vi "GenerateTextFragments.vi"(8 "error in (no error)":errorcluster, 9 "textPosition in":u32, 10 "textFragment in":T1, 11 "xmlelement in":refnum<k20>) -> (0 "error out":errorcluster, 1 "textPosition out":u32, 2 "textFragments out":T1[](array[typedef]), 3 "xmlelement out":refnum<k20>)   [LabVIEW 2010, in "StyledText.lvlib"]
doc: "Generates text fragments from the given XML node. Uses recursion to read child nodes.\n\nCopyright (c) 2018, Martin Weiss\nAll rights reserved.\n\nRedistribution and use in source and binary forms, with or without modification, are permitted provided that the following conditions are met:\n\n1. Redistributions of source code must retain the above copyright notice, this list of conditions and the following disclaimer.\n\n2. Redistributions in binary form must reproduce the above copyright notice, this list of conditions and the following disclaimer in the documentation and/or other materials provided with the distribution.\n\nTHIS SOFTWARE IS PROVIDED BY THE COPYRIGHT HOLDERS AND CONTRIBUTORS \"AS IS\" AND ANY EXPRESS OR IMPLIED WARRANTIES, INCLUDING, BUT NOT LIMITED TO, THE IMPLIED WARRANTIES OF MERCHANTABILITY AND FITNESS FOR A PARTICULAR PURPOSE ARE DISCLAIMED. IN NO EVENT SHALL THE COPYRIGHT HOLDER OR CONTRIBUTORS BE LIABLE FOR ANY DIRECT, INDIRECT, INCIDENTAL, SPECIAL, EXEMPLARY, OR CONSEQUENTIAL DAMAGES (INCLUDING, BUT NOT LIMITED TO, PROCUREMENT OF SUBSTITUTE GOODS OR SERVICES; LOSS OF USE, DATA, OR PROFITS; OR BUSINESS INTERRUPTION) HOWEVER CAUSED AND ON ANY THEORY OF LIABILITY, WHETHER IN CONTRACT, STRICT LIABILITY, OR TORT (INCLUDING NEGLIGENCE OR OTHERWISE) ARISING IN ANY WAY OUT OF THE USE OF THIS SOFTWARE, EVEN IF ADVISED OF THE POSSIBILITY OF SUCH DAMAGE."
uses:
  StyledText.lvlib
  TextFragment.ctl
  <vilib>/Utility/miscctls.llb/LVSelectionTypeDef.ctl
  <vilib>/Utility/miscctls.llb/LVFontTypeDef.ctl
  <vilib>/xml/Close Reference(Node).vi
  Program Files (x86)/National Instruments/LabVIEW 2010/resource/objmgr/DOMUserDefRef.rc
  <vilib>/xml/NI_XML.lvlib
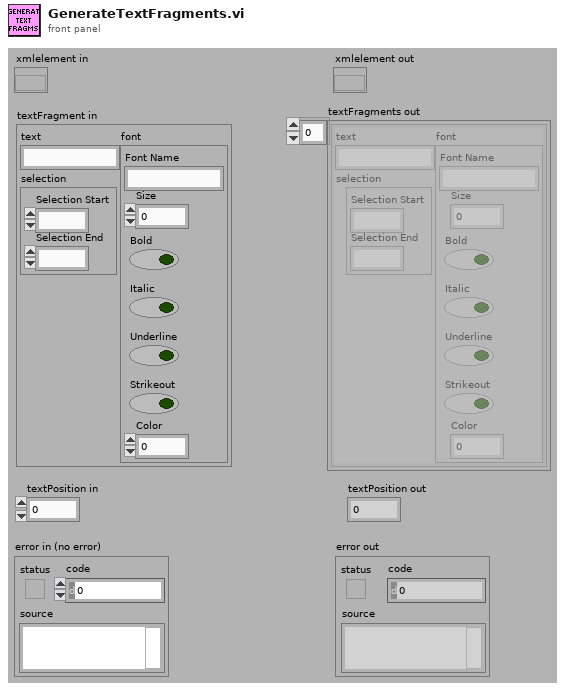
[diagram p1: front panel]
types:
  T1 = typedef "StyledText.lvlib/TextFragment.ctl" = cluster{"text":string, "selection":T2, "font":T3}
  T2 = typedef "LVSelectionTypeDef.ctl" = cluster{"Selection Start":u32, "Selection End":u32}
  T3 = typedef "LVFontTypeDef.ctl" = cluster{"Font Name":string, "Size":u16, "Bold":bool, "Italic":bool, "Underline":bool, "Strikeout":bool, "Color":u32}
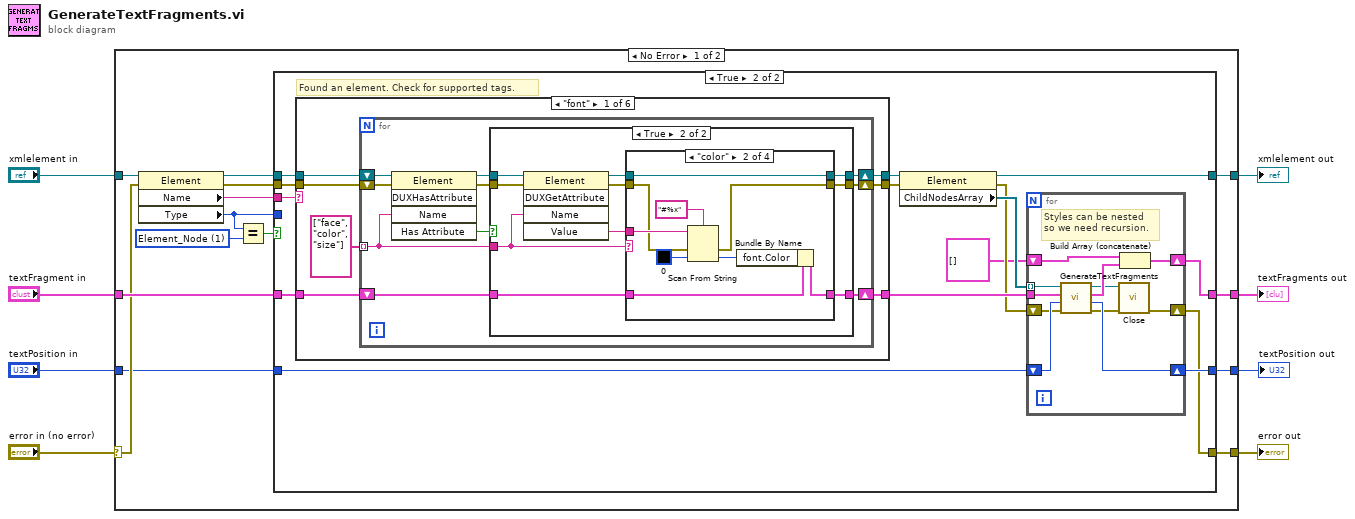
[diagram p0: block diagram]
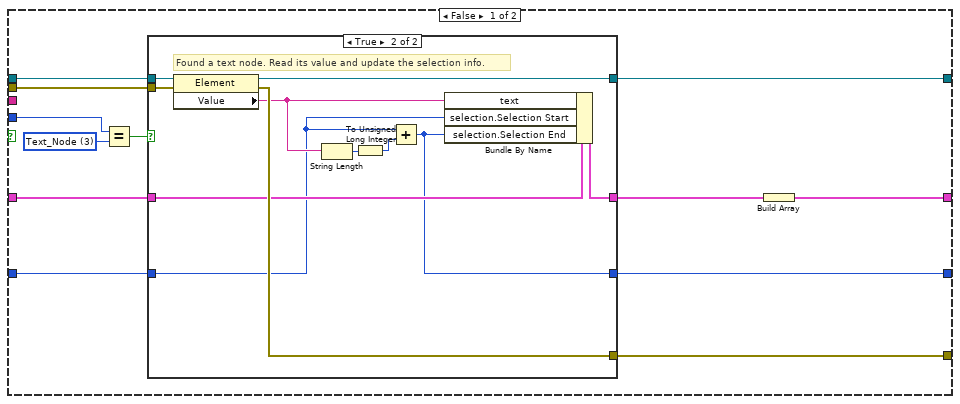
[diagram p2: hidden frame]
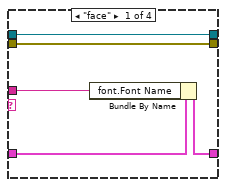
[diagram p5: hidden frame]
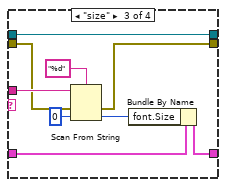
[diagram p6: hidden frame]
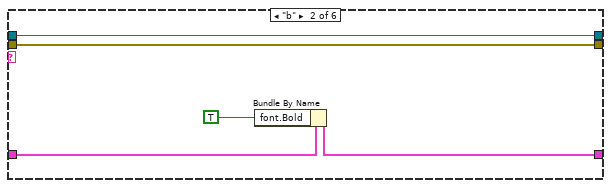
[diagram p8: hidden frame]
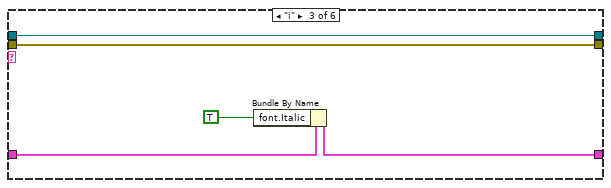
[diagram p9: hidden frame]
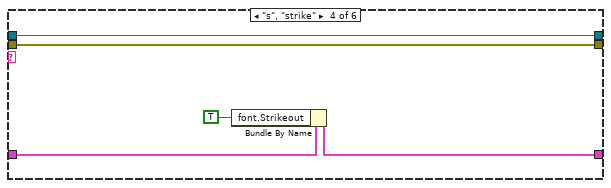
[diagram p10: hidden frame]
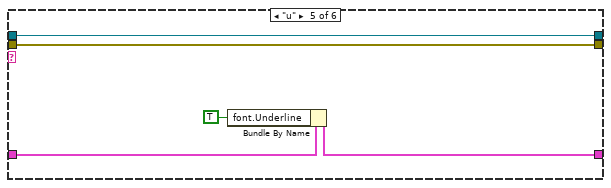
[diagram p11: hidden frame]
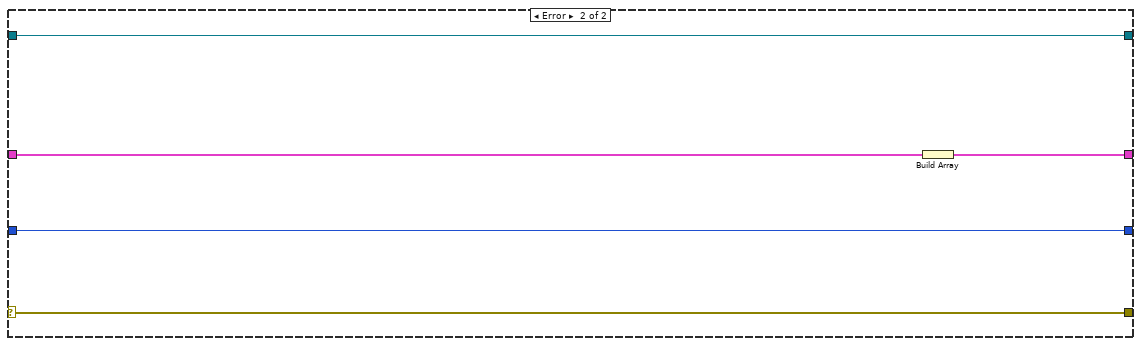
[diagram p13: hidden frame]
diagram:
  n1 = case shown="No Error" "error in (no error)" {
    selector: "error in (no error)" -> [w18 w158]
    tunnel: "textFragment in" -> [w22 w159]
    tunnel: [w21 w155] -> w7
    tunnel: "xmlelement in" -> [w20 w157]
    tunnel: [w15 w158] -> w4
    tunnel: [w11 w157] -> w3
    tunnel: "textPosition in" -> [w10 w156]
    tunnel: [w9 w156] -> w1
    frame No Error {
      w14 = 1 items=["Element_Node"=1, "Attribute_Node"=2, "Text_Node"=3, "CDATASection_Node"=4, "EntityReference_Node"=5, "Entity_Node"=6, "ProcessingInstruction_Node"=7, "Comment_Node"=8, "Document_Node"=9, "DocumentType_Node"=10, "DocumentFragment_Node"=11, "Notation_Node"=12] ("Node Type")
      n2 = property class="Element"(reference=w20, error in=w18) -> (reference out=w19:refnum<k20>, error out=w16:errorcluster, "Name"=w17:string, "Type"=w12:i32)
      n3 = Equal?(x=w12, y=w14) -> (x = y?=w13:bool)
      n4 = case shown="True" w13 {
        tunnel: w22 -> [w30 w64]
        tunnel: [w23 w52] -> w21
        tunnel: w19 -> [w31 w63]
        tunnel: w17 -> [_ w62]
        tunnel: w16 -> [w28 w61]
        tunnel: [w27 w50] -> w15
        tunnel: w12 -> [w33 _]
        tunnel: [w26 w59] -> w11
        tunnel: w10 -> [w25 w58]
        tunnel: [w24 w57] -> w9
        frame False {
          w34 = 3 items=["Element_Node"=1, "Attribute_Node"=2, "Text_Node"=3, "CDATASection_Node"=4, "EntityReference_Node"=5, "Entity_Node"=6, "ProcessingInstruction_Node"=7, "Comment_Node"=8, "Document_Node"=9, "DocumentType_Node"=10, "DocumentFragment_Node"=11, "Notation_Node"=12] ("Node Type")
          n5 = Equal?(x=w33, y=w34) -> (x = y?=w32:bool)
          n6 = case shown="True" w32 {
            tunnel: w31 -> [w36 w49]
            tunnel: w30 -> [w38 w44]
            tunnel: [w38 w43] -> w29
            tunnel: w28 -> [w37 w48]
            tunnel: [w37 w47] -> w27
            tunnel: [w36 w46] -> w26
            tunnel: w25 -> [w35 w42]
            tunnel: [w35 w41] -> w24
            frame False {
            }
            frame True {
              # "Found a text node. Read its value and update the selection info."
              n7 = property class="Element"(reference=w49, error in=w48) -> (reference out=w46:refnum<k20>, error out=w47:errorcluster, "Value"=w45:string)
              n8 = String Length(string=w45) -> (length=w40:i32)
              n9 = To Unsigned Long Integer(number=w40) -> (unsigned 32bit integer=w39:u32)
              n10 = Add(x=w42, y=w39) -> (x+y=w41:u32)
              n11 = Bundle By Name(cluster=w44, "text"=w45, "selection.Selection Start"=w42, "selection.Selection End"=w41) -> (w43:T1)
            }
          }
          n12 = Build Array(w29) -> (w23:T1[])
        }
        frame True {
          # "Found an element. Check for supported tags."
          n13 = case shown="\"font\"" w62 {
            tunnel: w63 -> [w78 w133 w138 w143 w148 w152]
            tunnel: [w82 w136 w141 w146 w151 w154] -> w60
            tunnel: w64 -> [w81 w134 w139 w144 w149 w154]
            tunnel: w61 -> [w80 w135 w140 w145 w150 w153]
            tunnel: [w79 w135 w140 w145 w150 w153] -> w55
            tunnel: [w77 w133 w138 w143 w148 w152] -> w56
            frame "font" {
              n14 = for {
                shift-right: [w87] -> w82
                shift-left: w81 -> [w86]
                shift-right: [w84] -> w79
                shift-left: w80 -> [w92]
                shift-right: [w85] -> w77
                shift-left: w78 -> [w90]
                tunnel: string[] ["face", "color", "size"] -> [w83] mode=indexing
                n15 = invoke class="Element" method="DUXHasAttribute"(reference=w90, error in=w92, "Name"=w83) -> (reference out=w89:refnum<k20>, error out=w91:errorcluster, "Has Attribute"=w88:bool)  [unwired: 2 in, 2 out]
                n16 = case shown="True" w88 {
                  tunnel: w91 -> [w94 w105]
                  tunnel: w89 -> [w95 w104]
                  tunnel: [w93 w102] -> w87
                  tunnel: w86 -> [w93 w101]
                  tunnel: [w95 w99] -> w85
                  tunnel: [w94 w97] -> w84
                  tunnel: w83 -> [_ w96]
                  frame False {
                  }
                  frame True {
                    n17 = invoke class="Element" method="DUXGetAttribute"(reference=w104, error in=w105, "Name"=w96) -> (reference out=w100:refnum<k20>, error out=w98:errorcluster, "Value"=w103:string)  [unwired: 2 in, 2 out]
                    n18 = case shown="\"color\"" w96 {
                      tunnel: [w109 w118 w127 w131] -> w102
                      tunnel: w101 -> [w110 w119 w128 w131]
                      tunnel: w100 -> [w107 w113 w122 w130]
                      tunnel: [w107 w113 w122 w130] -> w99
                      tunnel: w98 -> [w106 w112 w121 w129]
                      tunnel: [w106 w111 w120 w129] -> w97
                      tunnel: w103 -> [w108 w115 w125 _]
                      frame "face" {
                        n19 = Bundle By Name(cluster=w110, "font.Font Name"=w108) -> (w109:T1)
                      }
                      frame "color" {
                        n20 = Scan From String(format string="#%x", input string=w115, error in=w112, default 1=u32 0 ("color")) -> (error out=w111:errorcluster, output 1=w114:u32)  [unwired: 1 in, 2 out]
                        n21 = Bundle By Name(cluster=w119, "font.Color"=w114) -> (w118:T1)
                      }
                      frame "size" {
                        n22 = Scan From String(format string="%d", input string=w125, error in=w121, default 1=u16 0 ("default value 1")) -> (error out=w120:errorcluster, output 1=w124:u16)  [unwired: 1 in, 2 out]
                        n23 = Bundle By Name(cluster=w128, "font.Size"=w124) -> (w127:T1)
                      }
                      frame Default {
                      }
                    }
                  }
                }
              }
            }
            frame "b" {
              n24 = Bundle By Name(cluster=w134, "font.Bold"=TRUE) -> (w136:T1)
            }
            frame "i" {
              n25 = Bundle By Name(cluster=w139, "font.Italic"=TRUE) -> (w141:T1)
            }
            frame "s", "strike" {
              n26 = Bundle By Name(cluster=w144, "font.Strikeout"=TRUE) -> (w146:T1)
            }
            frame "u" {
              n27 = Bundle By Name(cluster=w149, "font.Underline"=TRUE) -> (w151:T1)
            }
            frame Default {
            }
          }
          n28 = property class="Element"(reference=w56, error in=w55) -> (reference out=w59:refnum<k20>, error out=w53:errorcluster, "ChildNodesArray"=w54:refnum<k20>[])
          n29 = for {
            tunnel: w60 -> [w75]
            tunnel: w54 -> [w72] mode=indexing
            shift-right: [w65] -> w50
            shift-left: w53 -> [w71]
            shift-right: [w73] -> w57
            shift-left: w58 -> [w74]
            shift-right: [w70] -> w52
            shift-left: T1[] [] -> [w69]
            # "Styles can be nested\nso we need recursion."
            n30 = call "GenerateTextFragments.vi"("error in (no error)"=w71, "textPosition in"=w74, "textFragment in"=w75, "xmlelement in"=w72) -> ("error out"=w66:errorcluster, "textPosition out"=w73:u32, "textFragments out"=w68:T1[], "xmlelement out"=w67:refnum<k20>)  [unwired: 4 in]
            n31 = call-poly <vilib>:"Close.vi"("error in (no error)"=w66, "node"=w67) -> ("error out"=w65:errorcluster)  [unwired: 7 in]
            n32 = Build Array (concatenate)(w69, w68) -> (w70:T1[])
          }
        }
      }
    }
    frame Error {
      n33 = Build Array(w159) -> (w155:T1[])
    }
  }
  "textFragments out" <- w7
  "error out" <- w4
  "xmlelement out" <- w3
  "textPosition out" <- w1
